vi "Sort Voltage.vi"(0 "Input Voltage":dbl[](array[numeric]), 5 "Output Voltage":dbl[](array[numeric])) -> (4 "Sorted Input Voltage":dbl[](array[numeric]), 6 "Sorted Output Voltage":dbl[](array[numeric]))   [LabVIEW 2020, in "LDO Dropout Voltage.lvlib"]
uses:
  LDO Dropout Voltage.lvlib
  b607da30-17c5-4249-b0c2-893b604dbd0f.vi
  <vilib>/Comparison/Less/Less Functor/Less Functor.lvclass
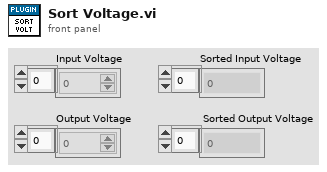
[diagram p1: front panel]
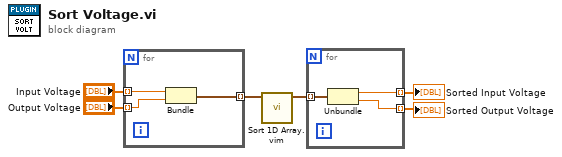
[diagram p0: block diagram]
diagram:
  n1 = for {
    tunnel: "Input Voltage" -> [w9] mode=indexing
    tunnel: "Output Voltage" -> [w8] mode=indexing
    tunnel: [w7] -> w5 mode=indexing
    n2 = Bundle("Numeric"=w9, "Numeric"=w8) -> (w7:cluster{"Numeric":dbl, "Numeric":dbl})  [unwired: 1 in]
  }
  n3 = call "Sort 1D Array.vim"("unsorted array"=w5) -> ("sorted array"=w6:cluster{"Numeric":dbl, "Numeric":dbl}[])  [unwired: 10 in]
  n4 = for {
    tunnel: w6 -> [w12] mode=indexing
    tunnel: [w11] -> w2 mode=indexing
    tunnel: [w10] -> w1 mode=indexing
    n5 = Unbundle(w12) -> ("Numeric"=w11:dbl, "Numeric"=w10:dbl)
  }
  "Sorted Input Voltage" <- w2
  "Sorted Output Voltage" <- w1
